vi "Sensor Compensation.vi"(4 "Init":T2, 5 "Joints":sgl[](array[numeric]), 6 "Sensor":T4 {"£nz" format="%.3f"; "£ny" format="%.3f"; "£nx" format="%.3f"; "Fz" format="%.2f"; "Fy" format="%.2f"; "Fx" format="%.2f"}, 7 "Add":bool) -> (0 "Weight (g)":dbl format="%.3f", 1 "theta(degree)":dbl format="%.3f", 2 "Compensation":T1 {"£nez" format="%.3f"; "£ney" format="%.3f"; "£nex" format="%.3f"; "Fez" format="%.2f"; "Fey" format="%.2f"; "Fex" format="%.2f"}, 3 "Record":T3 {"z" format="%.2f"; "G" format="%.3f"; "Mzo" format="%.3f"; "Myo" format="%.3f"; "Mxo" format="%.2f"; "Fzo" format="%.3f"; "Fyo" format="%.3f"; "Fxo" format="%.3f"; "£c" format="%.2f"; "y" format="%.2f"; "x" format="%.2f"})   [LabVIEW 2018]
uses:
  <vilib>/Analysis/Matrix/Datatypes/RealMatrix.ctl
  <vilib>/Analysis/_algsub.llb/Real PseudoInverse Matrix.vi
  <vilib>/Analysis/baseanly.llb/A x Vector.vi
  <vilib>/Analysis/Matrix/NI_Matrix.lvlib
  <vilib>/Analysis/NI_AALPro.lvlib
  <vilib>/Analysis/NI_AALBase.lvlib
panel:
  out "Count":u32
  out "Force arr":dbl[](array[numeric])
  out "Torque arr":dbl[](array[numeric])
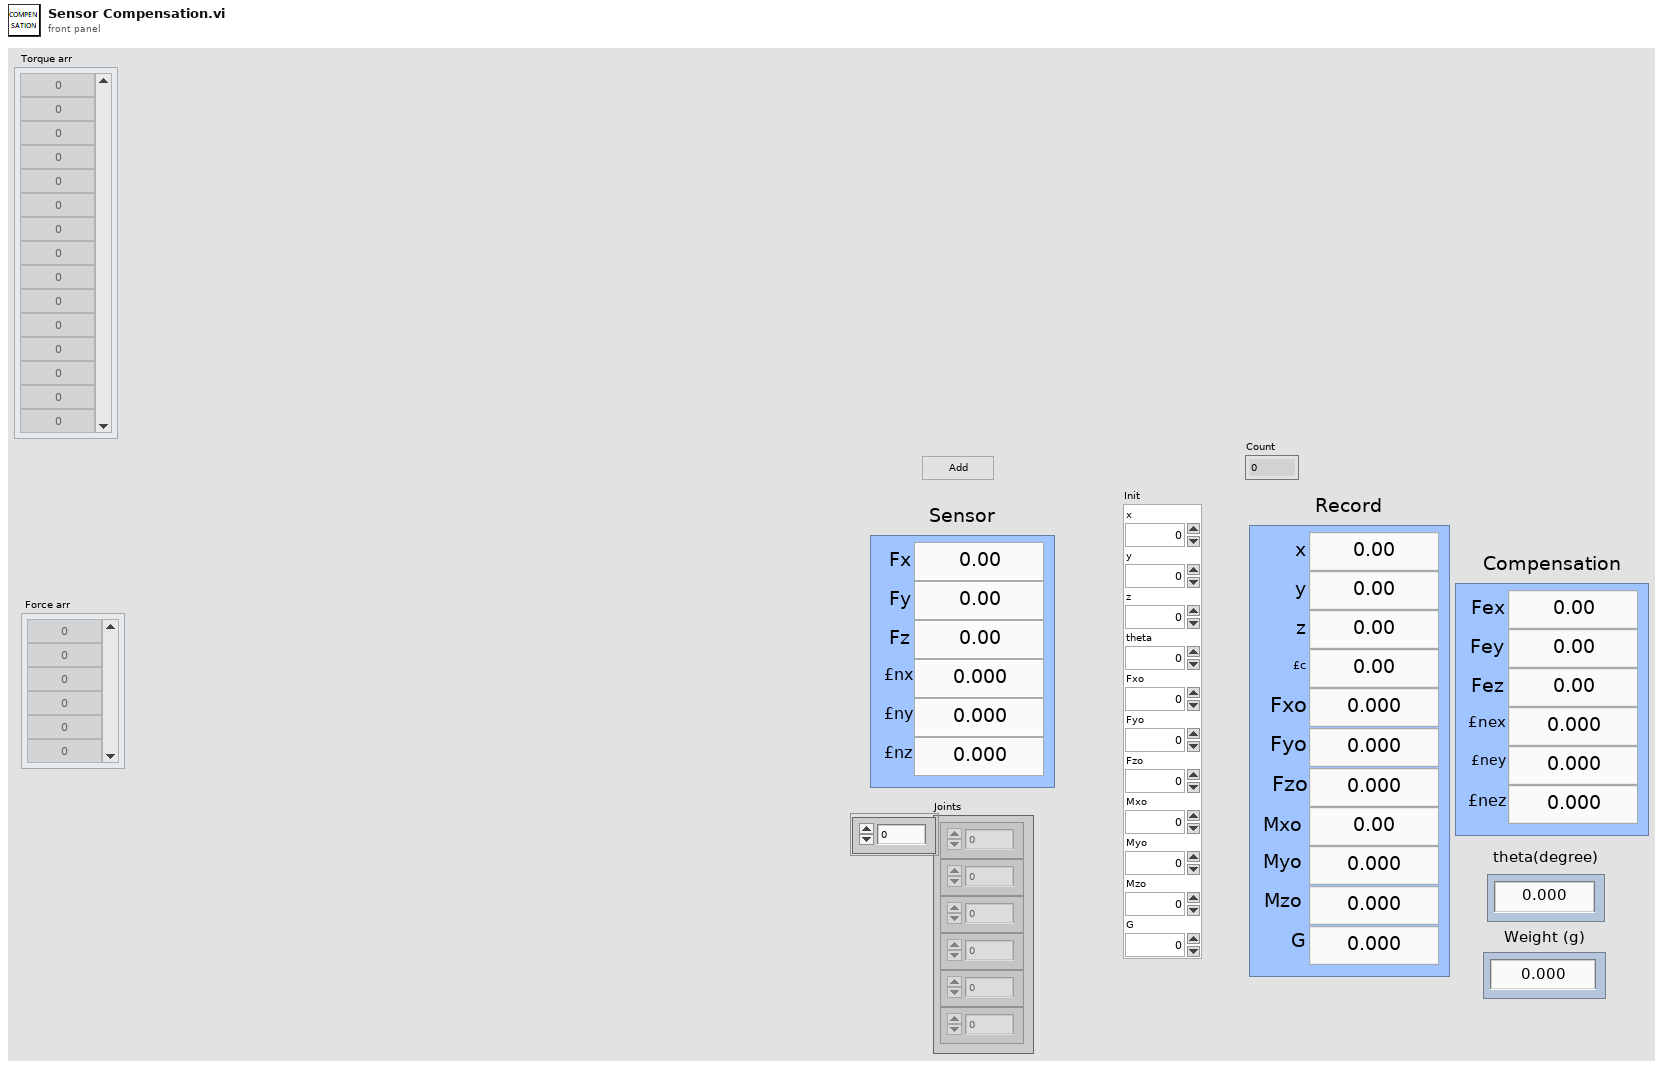
[diagram p1: front panel]
types:
  T1 = cluster{"Fex":dbl, "Fey":dbl, "Fez":dbl, " £nex":dbl, " £ney":dbl, " £nez":dbl}
  T2 = cluster{"x":dbl, "y":dbl, "z":dbl, "theta":dbl, "Fxo":dbl, "Fyo":dbl, "Fzo":dbl, "Mxo":dbl, "Myo":dbl, "Mzo":dbl, "G":dbl}
  T3 = cluster{"x":dbl, "y":dbl, "z":dbl, "£c":dbl, " Fxo":dbl, " Fyo":dbl, " Fzo":dbl, "Mxo":dbl, "Myo":dbl, "Mzo":dbl, "G":dbl}
  T4 = cluster{"Fx":dbl, "Fy":dbl, "Fz":dbl, " £nx":dbl, " £ny":dbl, " £nz":dbl}
  T5 = typedef "NI_Matrix.lvlib/RealMatrix.ctl" = dbl[][]
  T6 = cluster{dbl, dbl, dbl, dbl, dbl, dbl, dbl, dbl, dbl, dbl, dbl}
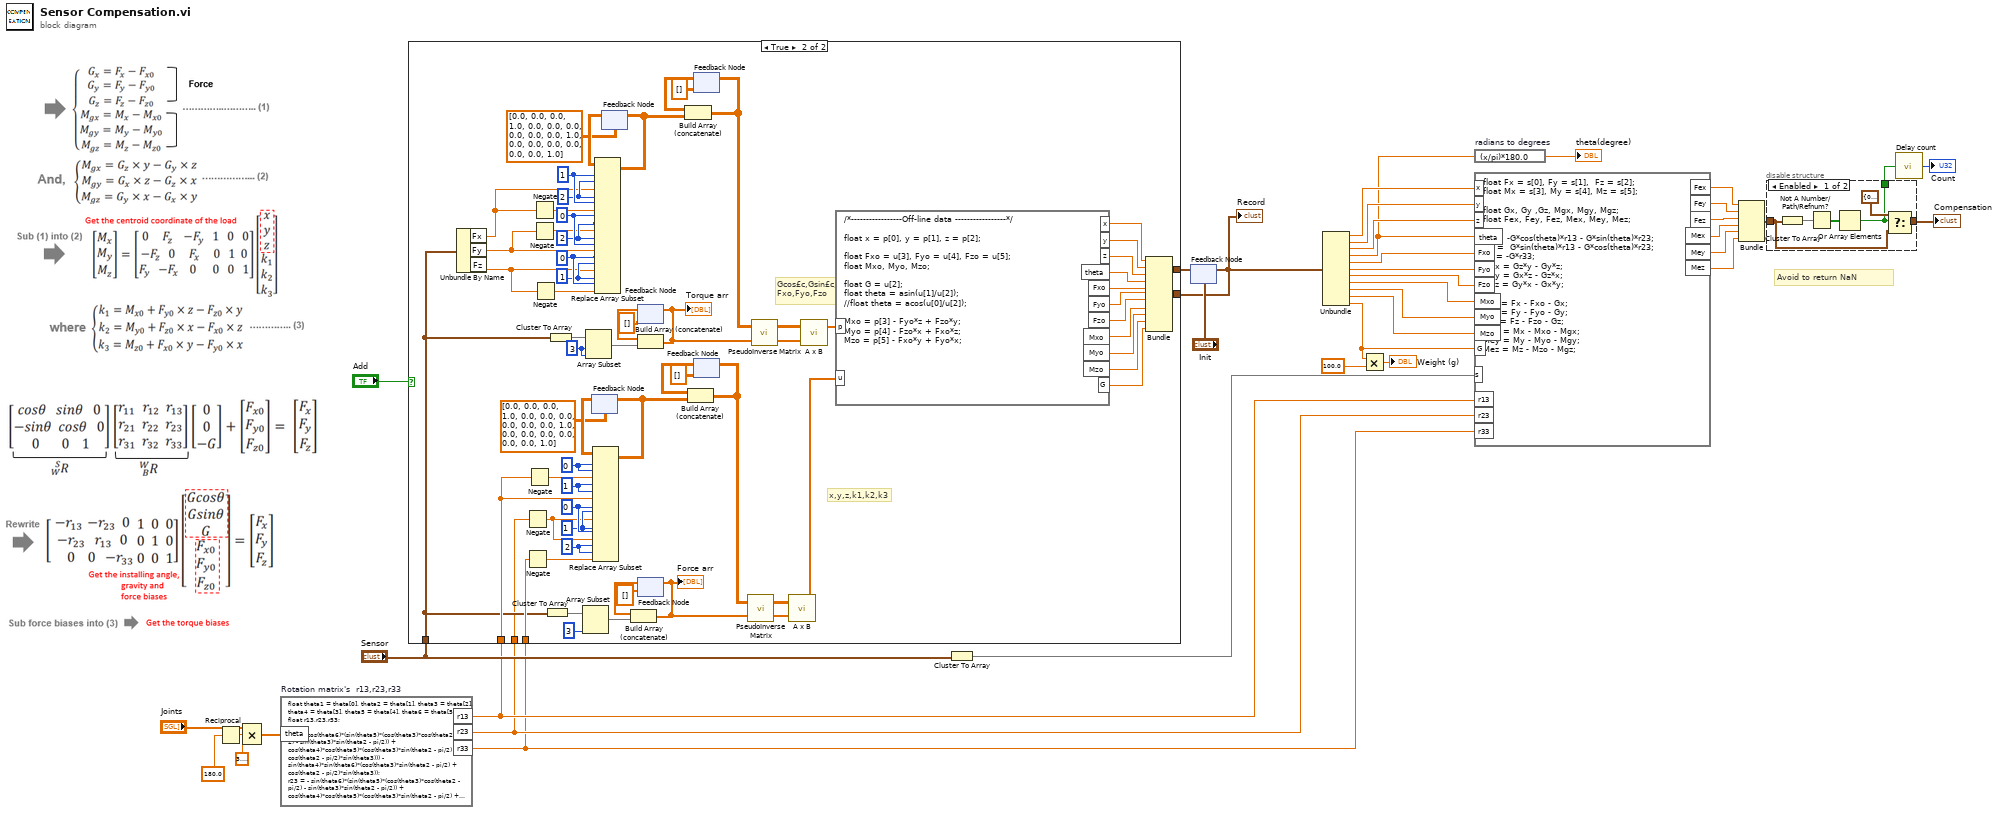
[diagram p0: block diagram]
diagram:
  # "Avoid to return NaN"
  n1 = Reciprocal(x=180.0 ("value")) -> (1/x=w35:dbl)
  n2 = Compound Arithmetic op=MULTIPLY("Joints", w35, 3.141592653589793) -> (w32:dbl[])
  n3 = formula code="float theta1 = theta[0], theta2 = theta[1], theta3 = theta[2], theta4 = theta[3], theta5 = theta[4], theta6 = theta[5];\nfloat r13,r23,r33;\n\nr13 = cos(theta6)*(sin(theta5)*(cos(theta3)*cos(theta2 - pi/2) - sin(theta3)*sin(theta2 - pi/2)) + cos(theta4)*cos(theta5)*(cos(theta3)*sin(theta2 - pi/2) + cos(theta2 - pi/2)*sin(theta3))) - sin(theta4)*sin(theta6)*(cos(theta3)*sin(theta2 - pi/2) + cos(theta2 - pi/2)*sin(theta3));\nr23 = - sin(theta6)*(sin(theta5)*(cos(theta3)*cos(theta2 - pi/2) - sin(theta3)*sin(theta2 - pi/2)) + cos(theta4)*cos(theta5)*(cos(theta3)*sin(theta2 - pi/2) + cos(theta2 - pi/2)*sin(theta3))) - cos(theta6)*sin(theta4)*(cos(theta3)*sin(theta2 - pi/2) + cos(theta2 - pi/2)*sin(theta3));\nr33 = cos(theta4)*sin(theta5)*(cos(theta3)*sin(theta2 - pi/2) + cos(theta2 - pi/2)*sin(theta3)) - cos(theta5)*(cos(theta3)*cos(theta2 - pi/2) - sin(theta3)*sin(theta2 - pi/2));" "Rotation matrix's  r13,r23,r33"("theta"=w32) -> ("r13"=w9:dbl, "r23"=w6:dbl, "r33"=w5:dbl)
  n4 = Cluster To Array(cluster="Sensor") -> (array=w10:dbl[])
  n5 = feedback #1("Init") -> (w38:T2)
  n6 = case shown="True" "Add" {
    tunnel: [w39 w90] -> w7
    tunnel: w9 -> [_ w51]
    tunnel: w5 -> [_ w50]
    tunnel: "Sensor" -> [_ w44]
    tunnel: w6 -> [_ w41]
    tunnel: w38 -> [w39 _]
    frame False {
    }
    frame True {
      w57 = 3 ("index")
      w63 = 1 ("disabled index (col)")
      w64 = 0 ("disabled index (row)")
      w65 = 2 ("disabled index (col)")
      w66 = 0 ("disabled index (row)")
      w67 = 2 ("disabled index (col)")
      w68 = 1 ("disabled index (row)")
      w83 = 2 ("disabled index (col)")
      w85 = 1 ("disabled index (col)")
      w77 = 1 ("disabled index (col)")
      w84 = 0 ("disabled index (col)")
      w86 = 0 ("disabled index (col)")
      # "x,y,z,k1,k2,k3"
      # "Gcos£c,Gsin£c,G,\nFxo,Fyo,Fzo"
      n7 = Unbundle By Name(w44) -> ("Fx"=w49:dbl, "Fy"=w48:dbl, "Fz"=w47:dbl)
      n8 = Negate(x=w41) -> (-x=w40:dbl)
      n9 = Negate(x=w50) -> (-x=w80:dbl)
      n10 = Negate(x=w51) -> (-x=w89:dbl)
      n11 = Negate(x=w49) -> (-x=w71:dbl)
      n12 = Negate(x=w48) -> (-x=w62:dbl)
      n13 = Negate(x=w47) -> (-x=w69:dbl)
      n14 = Cluster To Array(cluster=w44) -> (array=w43:dbl[])
      n15 = Cluster To Array(cluster=w44) -> (array=w46:dbl[])
      n16 = Array Subset(array=w43, length=3 ("index")) -> (w42:dbl[])  [unwired: 1 in]
      n17 = Array Subset(array=w46, index=w57, length=w57) -> (w45:dbl[])
      n18 = feedback #2(T5 [[0.0, 0.0, 0.0, 1.0, 0.0, 0.0], [0.0, 0.0, 0.0, 0.0, 1.0, 0.0], [0.0, 0.0, 0.0, 0.0, 0.0, 1.0]] ("Real Matrix")) -> (w88:T5)
      n19 = Replace Array Subset(array=w88, new element #1=w89, index (row) #1=w86, index (col) #1=w86, new element #2=w51, index (row) #2=w85, index (col) #2=w85, new element #3=w40, index (row) #3=w84, index (col) #3=w77, new element #4=w40, index (row) #4=w77, index (col) #4=w84, new element #5=w80, index (row) #5=w83, index (col) #5=w83) -> (w79:T5)
      n20 = feedback-in #2(w79) -> ()
      n21 = feedback #3(T5 [[0.0, 0.0, 0.0, 1.0, 0.0, 0.0], [0.0, 0.0, 0.0, 0.0, 1.0, 0.0], [0.0, 0.0, 0.0, 0.0, 0.0, 1.0]] ("Real Matrix")) -> (w70:T5)
      n22 = Replace Array Subset(array=w70, new element #1=w49, index (row) #1=w68, index (col) #1=w67, new element #2=w71, index (row) #2=w67, index (col) #2=w68, new element #3=w62, index (row) #3=w66, index (col) #3=w65, new element #4=w48, index (row) #4=w65, index (col) #4=w66, new element #5=w47, index (row) #5=w64, index (col) #5=w63, new element #6=w69, index (row) #6=w63, index (col) #6=w64) -> (w61:T5)
      n23 = feedback-in #3(w61) -> ()
      n24 = feedback #4(dbl[] []) -> (w56:dbl[])
      n25 = Build Array (concatenate)(w56, w45) -> (w52:dbl[])
      "Torque arr" <- w52
      n26 = feedback-in #4(w52) -> ()
      n27 = feedback #5(dbl[] []) -> (w74:dbl[])
      n28 = Build Array (concatenate)(w74, w42) -> (w76:dbl[])
      "Force arr" <- w76
      n29 = feedback-in #5(w76) -> ()
      n30 = feedback #6(T5 [] ("Real Matrix")) -> (w60:T5)
      n31 = Build Array (concatenate)(w60, w61) -> (w53:T5)
      n32 = feedback-in #6(w53) -> ()
      n33 = feedback #7(T5 [] ("Real Matrix")) -> (w72:T5)
      n34 = Build Array (concatenate)(w72, w79) -> (w78:T5)
      n35 = feedback-in #7(w78) -> ()
      n36 = call-poly <vilib>:"PseudoInverse Matrix.vi"("Input Matrix"=w78) -> ("PseudoInverse Matrix"=w82:T5)  [unwired: 1 in, 1 out]
      n37 = call-poly <vilib>:"PseudoInverse Matrix.vi"("Input Matrix"=w53) -> ("PseudoInverse Matrix"=w54:T5)  [unwired: 1 in, 1 out]
      n38 = call-poly <vilib>:"A x B.vi"("Vector"=w76, "A"=w82) -> ("A x Vector"=w102:dbl[])  [unwired: 1 out]
      n39 = call-poly <vilib>:"A x B.vi"("Vector"=w52, "A"=w54) -> ("A x Vector"=w103:dbl[])  [unwired: 1 out]
      n40 = formula code="/*-----------------Off-line data -----------------*/\n\nfloat x = p[0], y = p[1], z = p[2];\n\nfloat Fxo = u[3], Fyo = u[4], Fzo = u[5];\nfloat Mxo, Myo, Mzo;\n\nfloat G = u[2];\nfloat theta = asin(u[1]/u[2]); \n//float theta = acos(u[0]/u[2]); \n\nMxo = p[3] - Fyo*z + Fzo*y;\nMyo = p[4] - Fzo*x + Fxo*z;\nMzo = p[5] - Fxo*y + Fyo*x;"("p"=w103, "u"=w102) -> ("x"=w101:dbl, "y"=w100:dbl, "z"=w99:dbl, "theta"=w98:dbl, "Fxo"=w97:dbl, "Fyo"=w96:dbl, "Fzo"=w95:dbl, "Mxo"=w94:dbl, "Myo"=w93:dbl, "Mzo"=w92:dbl, "G"=w91:dbl)
      n41 = Bundle(w101, w100, w99, w98, w97, w96, w95, w94, w93, w92, w91) -> (w90:T6)  [unwired: 1 in]
    }
  }
  "Record" <- w7
  n42 = feedback-in #1(w7) -> ()
  n43 = Unbundle(w7) -> ("x"=w24:dbl, "y"=w23:dbl, "z"=w22:dbl, "theta"=w16:dbl, "Fxo"=w21:dbl, "Fyo"=w20:dbl, "Fzo"=w14:dbl, "Mxo"=w19:dbl, "Myo"=w18:dbl, "Mzo"=w17:dbl, "G"=w12:dbl)
  n44 = Multiply(x=w12, y=100.0 ("x")) -> (x*y=→"Weight (g)":dbl)
  n45 = expression code="(x/pi)*180.0" "radians to degrees"(w16) -> (→"theta(degree)":dbl)
  n46 = formula code="float Fx = s[0], Fy = s[1],  Fz = s[2];\nfloat Mx = s[3], My = s[4], Mz = s[5];\n\nfloat Gx, Gy ,Gz, Mgx, Mgy, Mgz;\nfloat Fex, Fey, Fez, Mex, Mey, Mez;\n\nGx = -G*cos(theta)*r13 - G*sin(theta)*r23;\nGy =  G*sin(theta)*r13 - G*cos(theta)*r23;\nGz = -G*r33;\nMgx = Gz*y - Gy*z;\nMgy = Gx*z - Gz*x;\nMgz = Gy*x - Gx*y;\n\nFex = Fx - Fxo - Gx;\nFey = Fy - Fyo - Gy;\nFez = Fz - Fzo - Gz;\nMex = Mx - Mxo - Mgx;\nMey = My - Myo - Mgy;\nMez = Mz - Mzo - Mgz;"("x"=w24, "y"=w23, "z"=w22, "theta"=w16, "Fxo"=w21, "Fyo"=w20, "Fzo"=w14, "Mxo"=w19, "Myo"=w18, "Mzo"=w17, "s"=w10, "G"=w12, "r13"=w9, "r23"=w6, "r33"=w5) -> ("Fex"=w30:dbl, "Fey"=w29:dbl, "Fez"=w28:dbl, "Mex"=w27:dbl, "Mey"=w26:dbl, "Mez"=w25:dbl)
  n47 = Bundle(w30, w29, w28, w27, w26, w25) -> (w3:cluster{dbl, dbl, dbl, dbl, dbl, dbl})  [unwired: 1 in]
  n48 = disable-structure shown="Enabled" {
    disable-tunnel: [w108 w110] -> w4
    disable-tunnel: w3 -> [w106 w110]
    disable-tunnel: [w104 _] -> w1
    frame Enabled {
      n49 = Cluster To Array ("Cluster To Array 2")(cluster=w106) -> (array=w109:dbl[])
      n50 = Not A Number/Path/Refnum?(number/path/refnum=w109) -> (NaN/Path/Refnum?=w105:bool[])
      n51 = Or Array Elements(Boolean array=w105) -> (logical OR=w104:bool)
      n52 = Select(t=cluster{dbl, dbl, dbl, dbl, dbl, dbl} {0.0, 0.0, 0.0, 0.0, 0.0, 0.0}, s=w104, f=w106) -> (s? t:f=w108:cluster{dbl, dbl, dbl, dbl, dbl, dbl})
    }
    frame Disabled {
    }
  }
  "Compensation" <- w4
  n53 = call "Delay count.vi"("Finished Late? [i-1]"=w1) -> ("Count"=→"Count":u32)
